vi "Write Context.vi"(8 "error in (no error)":errorcluster, 10 "Context":i32(ring)=1 items=["Formatting"=1, "Display"=2, "PreferredSize"=4, "RowDeletion"=8, "Parsing"=256, "Commit"=512, "InitialValueRestoration"=1024, "LeaveControl"=2048, "CurrentCellChange"=4096, "Scroll"=8192, "ClipboardContent"=16384], 11 "DataError in":refnum<class "DataError.lvclass">) -> (0 "error out":errorcluster, 3 "DataError out":refnum<class "DataError.lvclass">)   [LabVIEW 2016, in "DataGrid.lvlib" / "DataError.lvclass"]
uses:
  <userlib>/LabVIEWdotNetDataGrid/source/Events/DataError/DataError.lvclass
  <userlib>/LabVIEWdotNetDataGrid/source/Events/DataError/DataError.lvclass/DataError.ctl
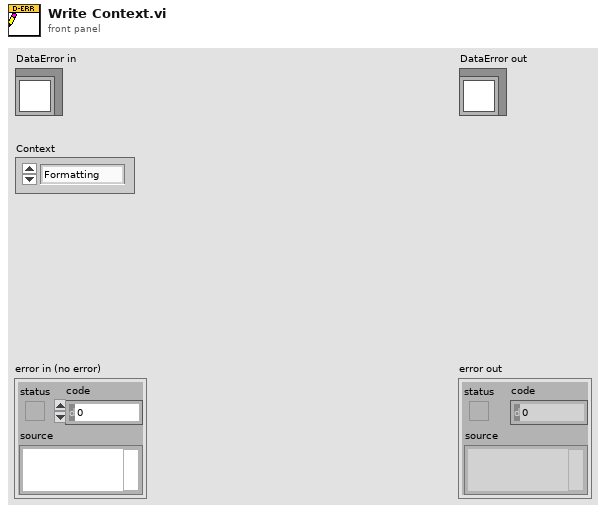
[diagram p1: front panel]
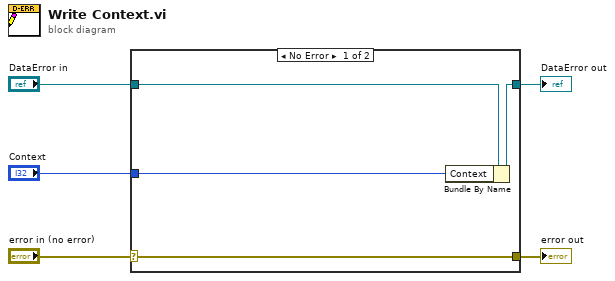
[diagram p0: block diagram]
diagram:
  n1 = case shown="No Error" "error in (no error)" {
    selector: "error in (no error)" -> [w9 w10]
    tunnel: [w9 w10] -> w4
    tunnel: [w7 w11] -> w2
    tunnel: "DataError in" -> [w8 w11]
    tunnel: "Context" -> [w6 _]
    frame No Error {
      n2 = Bundle By Name(cluster=w8, "Context"=w6) -> (w7:refnum<class "DataError.lvclass">)
    }
    frame Error {
    }
  }
  "error out" <- w4
  "DataError out" <- w2
